vi "JKISM++ Make String Argument Safe.vi"(2 "Argurment String":string="eaasdf->fqwvrf") -> (7 "Safe Argurment String":string)   [LabVIEW 2014, in "JKI State Machine++.lvlib"]
uses:
  JKI State Machine++.lvlib
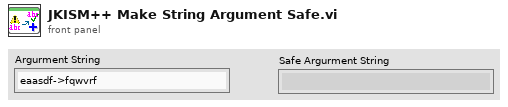
[diagram p1: front panel]
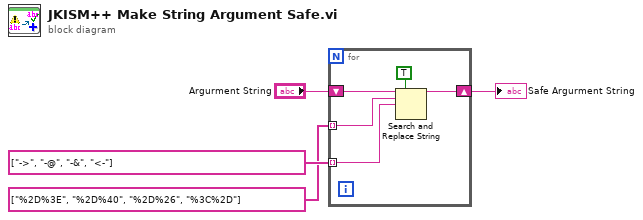
[diagram p0: block diagram]
diagram:
  n1 = for {
    shift-right: [w7] -> w3
    shift-left: "Argurment String" -> [w9]
    tunnel: string[] ["%2D%3E", "%2D%40", "%2D%26", "%3C%2D"] -> [w6] mode=indexing
    tunnel: string[] ["->", "-@", "-&", "<-"] -> [w5] mode=indexing
    n2 = Search and Replace String(replace all?=TRUE ("replace all? (F)"), input string=w9, search string=w6, replace string=w5) -> (result string=w7:string)  [unwired: 4 in, 3 out]
  }
  "Safe Argurment String" <- w3
